vi "rsscope_core_global.vi"() -> ()   [LabVIEW 2014] (continued)
\n\nAvailable Repeated Capabilities:\nEyeDiagram: ED1, ED2, ED3, ED4\r\n\nRemote-control command(s):\nEYE<m>:HORizontal:ABSolute:POSition"}, {"Level"=5, "Class Only"=FALSE, "Identifier"="RSSCOPE_ATTR_EYE_DIAGRAM_HORIZONTAL_SETTINGS_BIT_RATE", "Descriptive Name"="Eye Diagram Horizontal Settings Bit Rate", "Data Type"=1, "Command"="EYE{EyeDiagram}:HOR:UINT:BITR", "Access"=2, "Range Table"="RsScope_rngEyeDiagramHorizontalSettingsBitRate", "Read Callback"="", "Write Callback"="", "Supported Models"="", "Instrument Options"="K91|K93", "Flags"=0, "Help"="Sets the nominal frequency or bit rate of the data signal.\n\nAvailable Repeated Capabilities:\nEyeDiagram: ED1, ED2, ED3, ED4\r\n\nRemote-control command(s):\nEYE<m>:HORizontal:UINTerval:BITRate"}, {"Level"=5, "Class Only"=FALSE, "Identifier"="RSSCOPE_ATTR_EYE_DIAGRAM_HORIZONTAL_SETTINGS_RANGE_UI", "Descriptive Name"="Eye Diagram Horizontal Settings Range UI", "Data Type"=1, "Command"="EYE{EyeDiagram}:HOR:UINT:RANG", "Access"=2, "Range Table"="RsScope_rngEyeDiagramHorizontalSettingsRangeUI", "Read Callback"="", "Write Callback"="", "Supported Models"="", "Instrument Options"="K91|K93", "Flags"=0, "Help"="Sets the number of unit intervals that are visible in the eye diagram.\n\nAvailable Repeated Capabilities:\nEyeDiagram: ED1, ED2, ED3, ED4\r\n\nRemote-control command(s):\nEYE<m>:HORizontal:UINTerval:RANGe"}, {"Level"=5, "Class Only"=FALSE, "Identifier"="RSSCOPE_ATTR_EYE_DIAGRAM_HORIZONTAL_SETTINGS_POSITION_UI", "Descriptive Name"="Eye Diagram Horizontal Settings Position UI", "Data Type"=1, "Command"="EYE{EyeDiagram}:HOR:UINT:POS", "Access"=2, "Range Table"="RsScope_rngEyeDiagramHorizontalSettingsPositionUI", "Read Callback"="", "Write Callback"="", "Supported Models"="", "Instrument Options"="K91|K93", "Flags"=0, "Help"="Sets the zero point in the diagram, in unit intervals. The zero point is the alignment point on which the segment timestamps are superimposed.\n\nAvailable Repeated Capabilities:\nEyeDiagram: ED1, ED2, ED3, ED4\r\n\nRemote-control command(s):\nEYE<m>:HORizontal:UINTerval:POSition"}, {"Level"=4, "Class Only"=TRUE, "Identifier"="", "Descriptive Name"="Display", "Data Type"=0, "Command"="", "Access"=0, "Range Table"="", "Read Callback"="", "Write Callback"="", "Supported Models"="", "Instrument Options"="", "Flags"=0, "Help"="Define the appearance of the individual eye diagram."}, {"Level"=5, "Class Only"=FALSE, "Identifier"="RSSCOPE_ATTR_EYE_DIAGRAM_MAX_SLICES_PER_ACQUISITION", "Descriptive Name"="Eye Diagram Max Slices Per Acquisition", "Data Type"=0, "Command"="EYE{EyeDiagram}:MSL", "Access"=2, "Range Table"="RsScope_rngEyeDiagramMaxSlicesPerAcquisition", "Read Callback"="", "Write Callback"="", "Supported Models"="", "Instrument Options"="K91|K93", "Flags"=0, "Help"="Sets the number of waveform slices for a single acquisition.\n\nAvailable Repeated Capabilities:\nEyeDiagram: ED1, ED2, ED3, ED4\r\n\nRemote-control command(s):\nEYE<m>:MSLices"}, {"Level"=5, "Class Only"=FALSE, "Identifier"="RSSCOPE_ATTR_EYE_DIAGRAM_EYE_STRIPE_DISPLAY_MODE", "Descriptive Name"="Eye Diagram Eye Stripe Display Mode", "Data Type"=0, "Command"="EYE{EyeDiagram}:DISP", "Access"=2, "Range Table"="RsScope_rngEyeDiagramEyeStripeDisplayMode", "Read Callback"="", "Write Callback"="", "Supported Models"="", "Instrument Options"="K91|K93", "Flags"=0, "Help"="Defines when the eye stripe is shown: always, never, or during mask tests.\n\nAvailable Repeated Capabilities:\nEyeDiagram: ED1, ED2, ED3, ED4\r\n\nRemote-control command(s):\nEYE<m>:DISPlay[:MODE]"}, {"Level"=4, "Class Only"=TRUE, "Identifier"="", "Descriptive Name"="Qualify", "Data Type"=0, "Command"="", "Access"=0, "Range Table"="", "Read Callback"="", "Write Callback"="", "Supported Models"="", "Instrument Options"="", "Flags"=0, "Help"="Restrict the slices that contribute to the eye diagram. The restriction can be in horizontal direction (gate), or in vertical direction using the reference level."}, {"Level"=5, "Class Only"=FALSE, "Identifier"="RSSCOPE_ATTR_EYE_DIAGRAM_GATE_STATE", "Descriptive Name"="Eye Diagram Gate State", "Data Type"=3, "Command"="EYE{EyeDiagram}:QUAL:GATE", "Access"=2, "Range Table"="", "Read Callback"="", "Write Callback"="", "Supported Models"="", "Instrument Options"="K91|K93", "Flags"=0, "Help"="Enables the gate.\n\nAvailable Repeated Capabilities:\nEyeDiagram: ED1, ED2, ED3, ED4\r\n\nRemote-control command(s):\nEYE<m>:QUALify:GATE[:STATe]"}, {"Level"=5, "Class Only"=FALSE, "Identifier"="RSSCOPE_ATTR_EYE_DIAGRAM_GATE_COUPLING_MODE", "Descriptive Name"="Eye Diagram Gate Coupling Mode", "Data Type"=0, "Command"="EYE{EyeDiagram}:QUAL:GATE:COUP", "Access"=2, "Range Table"="RsScope_rngEyeDiagramGateCouplingMode", "Read Callback"="", "Write Callback"="", "Supported Models"="", "Instrument Options"="K91|K93", "Flags"=0, "Help"="Sets the gate coupling. To use cursor lines or zoom areas as gate limits, the cursor or zoom must be defined before.\n\nAvailable Repeated Capabilities:\nEyeDiagram: ED1, ED2, ED3, ED4\r\n\nRemote-control command(s):\nEYE<m>:QUALify:GATE:COUPling"}, {"Level"=5, "Class Only"=FALSE, "Identifier"="RSSCOPE_ATTR_EYE_DIAGRAM_GATE_MODE", "Descriptive Name"="Eye Diagram Gate Mode", "Data Type"=0, "Command"="EYE{EyeDiagram}:QUAL:GATE:MODE", "Access"=2, "Range Table"="rsscope_rngAbsRel", "Read Callback"="", "Write Callback"="", "Supported Models"="", "Instrument Options"="K91|K93", "Flags"=0, "Help"="Defines whether the gate limit is defined in absolute or relative values when no gate coupling is set.\n\nAvailable Repeated Capabilities:\nEyeDiagram: ED1, ED2, ED3, ED4\r\n\nRemote-control command(s):\nEYE<m>:QUALify:GATE:MODE"}, {"Level"=5, "Class Only"=FALSE, "Identifier"="RSSCOPE_ATTR_EYE_DIAGRAM_GATE_ABSOLUTE_START", "Descriptive Name"="Eye Diagram Gate Absolute Start", "Data Type"=1, "Command"="EYE{EyeDiagram}:QUAL:GATE:ABS:STAR", "Access"=2, "Range Table"="", "Read Callback"="", "Write Callback"="", "Supported Models"="", "Instrument Options"="K91|K93", "Flags"=0, "Help"="Set the absolute time values for gate start.\n\nAvailable Repeated Capabilities:\nEyeDiagram: ED1, ED2, ED3, ED4\r\n\nRemote-control command(s):\nEYE<m>:QUALify:GATE:ABSolute:STARt"}, {"Level"=5, "Class Only"=FALSE, "Identifier"="RSSCOPE_ATTR_EYE_DIAGRAM_GATE_ABSOLUTE_STOP", "Descriptive Name"="Eye Diagram Gate Absolute Stop", "Data Type"=1, "Command"="EYE{EyeDiagram}:QUAL:GATE:ABS:STOP", "Access"=2, "Range Table"="", "Read Callback"="", "Write Callback"="", "Supported Models"="", "Instrument Options"="K91|K93", "Flags"=0, "Help"="Set the absolute time values for gate end.\n\nAvailable Repeated Capabilities:\nEyeDiagram: ED1, ED2, ED3, ED4\r\n\nRemote-control command(s):\nEYE<m>:QUALify:GATE:ABSolute:STOP"}, {"Level"=5, "Class Only"=FALSE, "Identifier"="RSSCOPE_ATTR_EYE_DIAGRAM_GATE_RELATIVE_START", "Descriptive Name"="Eye Diagram Gate Relative Start", "Data Type"=1, "Command"="EYE{EyeDiagram}:QUAL:GATE:REL:STAR", "Access"=2, "Range Table"="RsScope_rngPercent", "Read Callback"="", "Write Callback"="", "Supported Models"="", "Instrument Options"="K91|K93", "Flags"=0, "Help"="Set the relative values for gate start and gate end.\n\nAvailable Repeated Capabilities:\nEyeDiagram: ED1, ED2, ED3, ED4\r\n\nRemote-control command(s):\nEYE<m>:QUALify:GATE:RELative:STARt"}, {"Level"=5, "Class Only"=FALSE, "Identifier"="RSSCOPE_ATTR_EYE_DIAGRAM_GATE_RELATIVE_STOP", "Descriptive Name"="Eye Diagram Gate Relative Stop", "Data Type"=1, "Command"="EYE{EyeDiagram}:QUAL:GATE:REL:STOP", "Access"=2, "Range Table"="RsScope_rngPercent", "Read Callback"="", "Write Callback"="", "Supported Models"="", "Instrument Options"="K91|K93", "Flags"=0, "Help"="Set the relative values for gate start and gate end.\n\nAvailable Repeated Capabilities:\nEyeDiagram: ED1, ED2, ED3, ED4\r\n\nRemote-control command(s):\nEYE<m>:QUALify:GATE:RELative:STOP"}, {"Level"=5, "Class Only"=FALSE, "Identifier"="RSSCOPE_ATTR_EYE_DIAGRAM_GATE_CURSOR", "Descriptive Name"="Eye Diagram Gate Cursor", "Data Type"=0, "Command"="EYE{EyeDiagram}:QUAL:GATE:CURS", "Access"=2, "Range Table"="rsscope_rngCursor", "Read Callback"="", "Write Callback"="", "Supported Models"="", "Instrument Options"="K91|K93", "Flags"=0, "Help"="Selects the cursor set to be used for eye gating. The gate area is defined by the cursor lines.\n\nAvailable Repeated Capabilities:\nEyeDiagram: ED1, ED2, ED3, ED4\r\n\nRemote-control command(s):\nEYE<m>:QUALify:GATE:CURSor"}, {"Level"=5, "Class Only"=FALSE, "Identifier"="RSSCOPE_ATTR_EYE_DIAGRAM_SIGNAL_STATE", "Descriptive Name"="Eye Diagram Signal State", "Data Type"=3, "Command"="EYE{EyeDiagram}:QUAL:SIGN", "Access"=2, "Range Table"="", "Read Callback"="", "Write Callback"="", "Supported Models"="", "Instrument Options"="K91|K93", "Flags"=0, "Help"="Enables the waveform-based qualification for the eye generation.\n\nAvailable Repeated Capabilities:\nEyeDiagram: ED1, ED2, ED3, ED4\r\n\nRemote-control command(s):\nEYE<m>:QUALify:SIGNal[:STATe]"}, {"Level"=5, "Class Only"=FALSE, "Identifier"="RSSCOPE_ATTR_EYE_DIAGRAM_SIGNAL_SOURCE", "Descriptive Name"="Eye Diagram Signal Source", "Data Type"=0, "Command"="EYE{EyeDiagram}:QUAL:SIGN:SOUR", "Access"=2, "Range Table"="rsscope_rngEyeDiagramSource", "Read Callback"="", "Write Callback"="", "Supported Models"="", "Instrument Options"="K91|K93", "Flags"=0, "Help"="Selects the waveform to be compared.\n\nAvailable Repeated Capabilities:\nEyeDiagram: ED1, ED2, ED3, ED4\r\n\nRemote-control command(s):\nEYE<m>:QUALify:SIGNal:SOURce"}, {"Level"=5, "Class Only"=FALSE, "Identifier"="RSSCOPE_ATTR_EYE_DIAGRAM_SIGNAL_CONDITION", "Descriptive Name"="Eye Diagram Signal Condition", "Data Type"=0, "Command"="EYE{EyeDiagram}:QUAL:SIGN:COND", "Access"=2, "Range Table"="rsscope_rngEyeDiagramSignalCondition", "Read Callback"="", "Write Callback"="", "Supported Models"="", "Instrument Options"="K91|K93", "Flags"=0, "Help"="Selects the comparison condition: the waveform level must be greater or less than the threshold.\n\nAvailable Repeated Capabilities:\nEyeDiagram: ED1, ED2, ED3, ED4\r\n\nRemote-control command(s):\nEYE<m>:QUALify:SIGNal:CONDition"}, {"Level"=5, "Class Only"=FALSE, "Identifier"="RSSCOPE_ATTR_EYE_DIAGRAM_SIGNAL_VERTICAL_REFERENCE_LEVEL", "Descriptive Name"="Eye Diagram Signal Vertical Reference Level", "Data Type"=0, "Command"="EYE{EyeDiagram}:QUAL:SIGN:LSEL", "Access"=2, "Range Table"="RsScope_rngEyeDiagramVerticalReferenceLevel", "Read Callback"="", "Write Callback"="", "Supported Models"="", "Instrument Options"="K91|K93", "Flags"=0, "Help"="Selects the threshold. You can use the lower, middle, or upper reference level. These levels are the reference levels that are defined for measurements.\n\nAvailable Repeated Capabilities:\nEyeDiagram: ED1, ED2, ED3, ED4\r\n\nRemote-control command(s):\nEYE<m>:QUALify:SIGNal:LSELect"}, {"Level"=4, "Class Only"=TRUE, "Identifier"="", "Descriptive Name"="Filter", "Data Type"=0, "Command"="", "Access"=0, "Range Table"="", "Read Callback"="", "Write Callback"="", "Supported Models"="", "Instrument Options"="", "Flags"=0, "Help"="Select waveform slices for eye generation dependent on the bit status."}, {"Level"=5, "Class Only"=FALSE, "Identifier"="RSSCOPE_ATTR_EYE_DIAGRAM_FILTER_STATE", "Descriptive Name"="Eye Diagram Filter State", "Data Type"=3, "Command"="EYE{EyeDiagram}:FILT:STAT", "Access"=2, "Range Table"="", "Read Callback"="", "Write Callback"="", "Supported Models"="", "Instrument Options"="K91|K93", "Flags"=0, "Help"="Applies the filter settings to the data signal.\n\nAvailable Repeated Capabilities:\nEyeDiagram: ED1, ED2, ED3, ED4\r\n\nRemote-control command(s):\nEYE<m>:FILTer:STATe"}, {"Level"=5, "Class Only"=FALSE, "Identifier"="RSSCOPE_ATTR_EYE_DIAGRAM_FILTER_BIT_SEQUENCE_MODE", "Descriptive Name"="Eye Diagram Filter Bit Sequence Mode", "Data Type"=0, "Command"="EYE{EyeDiagram}:FILT:BPAT:MODE", "Access"=2, "Range Table"="RsScope_rngEyeDiagramFilterBitSequenceMode", "Read Callback"="", "Write Callback"="", "Supported Models"="", "Instrument Options"="K91|K93", "Flags"=0, "Help"="Selects which bits contribute to the eye generation.\n\nAvailable Repeated Capabilities:\nEyeDiagram: ED1, ED2, ED3, ED4\r\n\nRemote-control command(s):\nEYE<m>:FILTer:BPATtern:MODE"}, {"Level"=5, "Class Only"=FALSE, "Identifier"="RSSCOPE_ATTR_EYE_DIAGRAM_FILTER_PATTERN_CENTER_BIT", "Descriptive Name"="Eye Diagram Filter Pattern Center Bit", "Data Type"=0, "Command"="EYE{EyeDiagram}:FILT:BPAT:CENT", "Access"=2, "Range Table"="RsScope_rngBitState", "Read Callback"="", "Write Callback"="", "Supported Models"="", "Instrument Options"="K91|K93", "Flags"=0, "Help"="Set the values of the indicated center bits.\n\nAvailable Repeated Capabilities:\nEyeDiagram: ED1, ED2, ED3, ED4\r\n\nRemote-control command(s):\nEYE<m>:FILTer:BPATtern:CENTer"}, {"Level"=5, "Class Only"=FALSE, "Identifier"="RSSCOPE_ATTR_EYE_DIAGRAM_FILTER_PATTERN_SHIFT_BIT_LEFT", "Descriptive Name"="Eye Diagram Filter Pattern Shift Bit Left", "Data Type"=4, "Command"="EYE{EyeDiagram}:FILT:BPAT:SLEF", "Access"=1, "Range Table"="", "Read Callback"="", "Write Callback"="", "Supported Models"="", "Instrument Options"="K91|K93", "Flags"=0, "Help"="Shifts the pattern one bit to the left.\n\nAvailable Repeated Capabilities:\nEyeDiagram: ED1, ED2, ED3, ED4\r\n\nRemote-control command(s):\nEYE<m>:FILTer:BPATtern:SLEFt"}, {"Level"=5, "Class Only"=FALSE, "Identifier"="RSSCOPE_ATTR_EYE_DIAGRAM_FILTER_PATTERN_SHIFT_BIT_RIGHT", "Descriptive Name"="Eye Diagram Filter Pattern Shift Bit Right", "Data Type"=4, "Command"="EYE{EyeDiagram}:FILT:BPAT:SRIG", "Access"=1, "Range Table"="", "Read Callback"="", "Write Callback"="", "Supported Models"="", "Instrument Options"="K91|K93", "Flags"=0, "Help"="Shifts the pattern one bit to the right.\n\nAvailable Repeated Capabilities:\nEyeDiagram: ED1, ED2, ED3, ED4\r\n\nRemote-control command(s):\nEYE<m>:FILTer:BPATtern:SRIGht"}, {"Level"=5, "Class Only"=FALSE, "Identifier"="RSSCOPE_ATTR_EYE_DIAGRAM_FILTER_FRAME_TYPE", "Descriptive Name"="Eye Diagram Filter Frame Type", "Data Type"=0, "Command"="EYE{EyeDiagram}:FILT:DDR:FTYP", "Access"=2, "Range Table"="RsScope_rngEyeDiagramDDRFrameFilter", "Read Callback"="", "Write Callback"="", "Supported Models"="", "Instrument Options"="K91|K93", "Flags"=0, "Help"="Sets which frame types contribute to the eye diagram.\n\nAvailable Repeated Capabilities:\nEyeDiagram: ED1, ED2, ED3, ED4\r\n\nRemote-control command(s):\nEYE<m>:FILTer:DDR:FTYPe"}, {"Level"=5, "Class Only"=FALSE, "Identifier"="RSSCOPE_ATTR_EYE_DIAGRAM_FILTER_LENGTH_ERRORS", "Descriptive Name"="Eye Diagram Filter Length Errors", "Data Type"=3, "Command"="EYE{EyeDiagram}:FILT:DDR:LEN", "Access"=2, "Range Table"="", "Read Callback"="", "Write Callback"="", "Supported Models"="", "Instrument Options"="K91|K93", "Flags"=0, "Help"="If enabled, the length errors contribute to the eye diagram.\n\nAvailable Repeated Capabilities:\nEyeDiagram: ED1, ED2, ED3, ED4\r\n\nRemote-control command(s):\nEYE<m>:FILTer:DDR:LENerror"}, {"Level"=5, "Class Only"=FALSE, "Identifier"="RSSCOPE_ATTR_EYE_DIAGRAM_FILTER_RESET", "Descriptive Name"="Eye Diagram Filter Reset", "Data Type"=4, "Command"="EYE{EyeDiagram}:FILT:BPAT:RES", "Access"=1, "Range Table"="", "Read Callback"="", "Write Callback"="", "Supported Models"="", "Instrument Options"="K91|K93", "Flags"=0, "Help"="Resets the bit sequence filter to the default (DC for all bits).\n\nAvailable Repeated Capabilities:\nEyeDiagram: ED1, ED2, ED3, ED4\r\n\nRemote-control command(s):\nEYE<m>:FILTer:BPATtern:RESet"}, {"Level"=4, "Class Only"=TRUE, "Identifier"="", "Descriptive Name"="Results of Mask Tests", "Data Type"=0, "Command"="", "Access"=0, "Range Table"="", "Read Callback"="", "Write Callback"="", "Supported Models"="", "Instrument Options"="", "Flags"=0, "Help"="Mask tests on eye diagrams"}, {"Level"=5, "Class Only"=FALSE, "Identifier"="RSSCOPE_ATTR_EYE_DIAGRAM_MASK_TESTS_SLICES_COMPLETED", "Descriptive Name"="Eye Diagram Mask Tests Slices Completed", "Data Type"=0, "Command"="MTES:RES:COUN:SLIC?", "Access"=0, "Range Table"="", "Read Callback"="rsscope_formatMaskNameInt32_ReadCallback.vi", "Write Callback"="", "Supported Models"="", "Instrument Options"="K91|K93", "Flags"=0, "Help"="Returns the number of slices that contributed to the eye diagram.\n\nAvailable Repeated Capabilities:\nNone\n\nRemote-control command(s):\nMTESt:RESult:COUNt:SLICes?"}, {"Level"=5, "Class Only"=FALSE, "Identifier"="RSSCOPE_ATTR_EYE_DIAGRAM_MASK_TESTS_SLICE_HITS", "Descriptive Name"="Eye Diagram Mask Tests Slice Hits", "Data Type"=0, "Command"="MTES:RES:COUN:FSL?", "Access"=0, "Range Table"="", "Read Callback"="rsscope_formatMaskNameInt32_ReadCallback.vi", "Write Callback"="", "Supported Models"="", "Instrument Options"="K91|K93", "Flags"=0, "Help"="Returns the number of slices that violated the mask.\n\nAvailable Repeated Capabilities:\nNone\n\nRemote-control command(s):\nMTESt:RESult:COUNt:FSLices?"}, {"Level"=5, "Class Only"=FALSE, "Identifier"="RSSCOPE_ATTR_EYE_DIAGRAM_MASK_TESTS_VIOLATION_INDEX", "Descriptive Name"="Eye Diagram Mask Tests Violation Index", "Data Type"=0, "Command"="", "Access"=2, "Range Table"="", "Read Callback"="", "Write Callback"="", "Supported Models"="", "Instrument Options"="K91|K93", "Flags"=0, "Help"="Sets selector repeated capability Violation. Corresponds to the number in the &apos;Violation&apos; column of mask test result.\n\nAvailable Repeated Capabilities:\nNone\n\nRemote-control command(s):\n"}, {"Level"=5, "Class Only"=FALSE, "Identifier"="RSSCOPE_ATTR_EYE_DIAGRAM_MASK_TESTS_VIOLATION_COUNT", "Descriptive Name"="Eye Diagram Mask Tests Violation Count", "Data Type"=0, "Command"="MTES:RES:VIOL<Violation>:COUN?", "Access"=0, "Range Table"="", "Read Callback"="rsscope_formatMaskNameViolationInt32_ReadCallback.vi", "Write Callback"="", "Supported Models"="", "Instrument Options"="K91|K93", "Flags"=0, "Help"="Returns the count of violations of mask test result.\n\nAvailable Repeated Capabilities:\nNone\n\nRemote-control command(s):\nMTESt:RESult:VIOLation<m>:COUNt?"}, {"Level"=5, "Class Only"=FALSE, "Identifier"="RSSCOPE_ATTR_EYE_DIAGRAM_MASK_TESTS_VIOLATION_START_TIME", "Descriptive Name"="Eye Diagram Mask Tests Violation Start Time", "Data Type"=1, "Command"="MTES:RES:VIOL<Violation>:STAR?", "Access"=0, "Range Table"="", "Read Callback"="rsscope_formatMaskNameViolationReal64_ReadCallback.vi", "Write Callback"="", "Supported Models"="", "Instrument Options"="K91|K93", "Flags"=0, "Help"="Return the start time of the slice with the indicated violation.\n\nAvailable Repeated Capabilities:\nNone\n\nRemote-control command(s):\nMTESt:RESult:VIOLation<m>:STARt?"}, {"Level"=5, "Class Only"=FALSE, "Identifier"="RSSCOPE_ATTR_EYE_DIAGRAM_MASK_TESTS_VIOLATION_STOP_TIME", "Descriptive Name"="Eye Diagram Mask Tests Violation Stop Time", "Data Type"=1, "Command"="MTES:RES:VIOL<Violation>:STOP?", "Access"=0, "Range Table"="", "Read Callback"="rsscope_formatMaskNameViolationReal64_ReadCallback.vi", "Write Callback"="", "Supported Models"="", "Instrument Options"="K91|K93", "Flags"=0, "Help"="Return the stop time of the slice with the indicated violation.\n\nAvailable Repeated Capabilities:\nNone\n\nRemote-control command(s):\nMTESt:RESult:VIOLation<m>:STOP?"}, {"Level"=5, "Class Only"=FALSE, "Identifier"="RSSCOPE_ATTR_EYE_DIAGRAM_MASK_TESTS_VIOLATION_SLICE", "Descriptive Name"="Eye Diagram Mask Tests Violation Slice", "Data Type"=0, "Command"="MTES:RES:VIOL<Violation>?", "Access"=0, "Range Table"="", "Read Callback"="rsscope_formatMaskNameViolationInt32_ReadCallback.vi", "Write Callback"="", "Supported Models"="", "Instrument Options"="K91|K93", "Flags"=0, "Help"="Returns the slice at the violation of mask test result.\n\nAvailable Repeated Capabilities:\nNone\n\nRemote-control command(s):\nMTESt:RESult:VIOLation<m>[:SLICe]?"}, {"Level"=2, "Class Only"=TRUE, "Identifier"="", "Descriptive Name"="100BASE-T1", "Data Type"=0, "Command"="", "Access"=0, "Range Table"="", "Read Callback"="", "Write Callback"="", "Supported Models"="", "Instrument Options"="", "Flags"=0, "Help"="This class contains attributes that configure the Ethernet protocol 100BASE-T1.\n\nAttributes in this class require option R&S RTO-K57."}, {"Level"=3, "Class Only"=FALSE, "Identifier"="RSSCOPE_ATTR_PROTOCOL_100BASE_T1_ATTENUATION", "Descriptive Name"="Protocol 100BASE-T1 Attenuation", "Data Type"=1, "Command"="BUS{SerialBus}:HBTO:ATTN", "Access"=2, "Range Table"="RsScope_rngProtocol100BASE_T1Attenuation", "Read Callback"="", "Write Callback"="", "Supported Models"="", "Instrument Options"="K57", "Flags"=0, "Help"="Sets the attenuation factor. It is used to de-amplify the reverse signal before subtracting it from the forward signal.\n\nAvailable Repeated Capabilities:\nSerialBus: SB1, SB2, SB3, SB4\r\n\nRemote-control command(s):\nBUS<m>:HBTO:ATTN"}, {"Level"=3, "Class Only"=FALSE, "Identifier"="RSSCOPE_ATTR_PROTOCOL_100BASE_T1_FORWARD_POSITIVE_SOURCE", "Descriptive Name"="Protocol 100BASE-T1 Forward Positive Source", "Data Type"=0, "Command"="BUS{SerialBus}:HBTO:FDAP", "Access"=2, "Range Table"="rsscope_rngProtocolDataSource", "Read Callback"="", "Write Callback"="", "Supported Models"="", "Instrument Options"="K57", "Flags"=0, "Help"="Selects the DA+ source of the provided forward single ended signal, if RSSCOPE_ATTR_PROTOCOL_100BASE_T1_FORWARD_SIGNAL_TYPE is set to Single.\n\nAvailable Repeated Capabilities:\nSerialBus: SB1, SB2, SB3, SB4\r\n\nRemote-control command(s):\nBUS<m>:HBTO:FDAP"}, {"Level"=3, "Class Only"=FALSE, "Identifier"="RSSCOPE_ATTR_PROTOCOL_100BASE_T1_FORWARD_NEGATIVE_SOURCE", "Descriptive Name"="Protocol 100BASE-T1 Forward Negative Source", "Data Type"=0, "Command"="BUS{SerialBus}:HBTO:FDAM", "Access"=2, "Range Table"="rsscope_rngProtocolDataSource", "Read Callback"="", "Write Callback"="", "Supported Models"="", "Instrument Options"="K57", "Flags"=0, "Help"="Selects the DA- source of the provided forward single ended signal, if RSSCOPE_ATTR_PROTOCOL_100BASE_T1_FORWARD_SIGNAL_TYPE is set to Single.\n\nAvailable Repeated Capabilities:\nSerialBus: SB1, SB2, SB3, SB4\r\n\nRemote-control command(s):\nBUS<m>:HBTO:FDAM"}, {"Level"=3, "Class Only"=FALSE, "Identifier"="RSSCOPE_ATTR_PROTOCOL_100BASE_T1_FORWARD_DIFFERENTIAL_SOURCE", "Descriptive Name"="Protocol 100BASE-T1 Forward Differential Source", "Data Type"=0, "Command"="BUS{SerialBus}:HBTO:FDIF", "Access"=2, "Range Table"="rsscope_rngProtocolDataSource", "Read Callback"="", "Write Callback"="", "Supported Models"="", "Instrument Options"="K57", "Flags"=0, "Help"="Sets the source of the provided forward differential signal, if RSSCOPE_ATTR_PROTOCOL_100BASE_T1_FORWARD_SIGNAL_TYPE is set to Differential.\n\nAvailable Repeated Capabilities:\nSerialBus: SB1, SB2, SB3, SB4\r\n\nRemote-control command(s):\nBUS<m>:HBTO:FDIF"}, {"Level"=3, "Class Only"=FALSE, "Identifier"="RSSCOPE_ATTR_PROTOCOL_100BASE_T1_FORWARD_SIGNAL_TYPE", "Descriptive Name"="Protocol 100BASE-T1 Forward Signal Type", "Data Type"=0, "Command"="BUS{SerialBus}:HBTO:FTYP", "Access"=2, "Range Table"="RsScope_rngSignalType", "Read Callback"="", "Write Callback"="", "Supported Models"="", "Instrument Options"="K57", "Flags"=0, "Help"="Sets the type of forward signal measurement.\n\nAvailable Repeated Capabilities:\nSerialBus: SB1, SB2, SB3, SB4\r\n\nRemote-control command(s):\nBUS<m>:HBTO:FTYP"}, {"Level"=3, "Class Only"=FALSE, "Identifier"="RSSCOPE_ATTR_PROTOCOL_100BASE_T1_REVERSE_POSITIVE_SOURCE", "Descriptive Name"="Protocol 100BASE-T1 Reverse Positive Source", "Data Type"=0, "Command"="BUS{SerialBus}:HBTO:RDAP", "Access"=2, "Range Table"="rsscope_rngProtocolDataSource", "Read Callback"="", "Write Callback"="", "Supported Models"="", "Instrument Options"="K57", "Flags"=0, "Help"="Selects the DA+ source of the provided reversed single ended signal, if RSSCOPE_ATTR_PROTOCOL_100BASE_T1_REVERSE_SIGNAL_TYPE is set to Single.\n\nAvailable Repeated Capabilities:\nSerialBus: SB1, SB2, SB3, SB4\r\n\nRemote-control command(s):\nBUS<m>:HBTO:RDAP"}, {"Level"=3, "Class Only"=FALSE, "Identifier"="RSSCOPE_ATTR_PROTOCOL_100BASE_T1_REVERSE_NEGATIVE_SOURCE", "Descriptive Name"="Protocol 100BASE-T1 Reverse Negative Source", "Data Type"=0, "Command"="BUS{SerialBus}:HBTO:RDAM", "Access"=2, "Range Table"="rsscope_rngProtocolDataSource", "Read Callback"="", "Write Callback"="", "Supported Models"="", "Instrument Options"="K57", "Flags"=0, "Help"="Selects the DA- source of the provided reversed single ended signal, if RSSCOPE_ATTR_PROTOCOL_100BASE_T1_REVERSE_SIGNAL_TYPE is set to Single.\n\nAvailable Repeated Capabilities:\nSerialBus: SB1, SB2, SB3, SB4\r\n\nRemote-control command(s):\nBUS<m>:HBTO:RDAM"}, {"Level"=3, "Class Only"=FALSE, "Identifier"="RSSCOPE_ATTR_PROTOCOL_100BASE_T1_REVERSE_DIFFERENTIAL_SOURCE", "Descriptive Name"="Protocol 100BASE-T1 Reverse Differential Source", "Data Type"=0, "Command"="BUS{SerialBus}:HBTO:RDIF", "Access"=2, "Range Table"="rsscope_rngProtocolDataSource", "Read Callback"="", "Write Callback"="", "Supported Models"="", "Instrument Options"="K57", "Flags"=0, "Help"="Sets the source of the provided reversed differential signal, if RSSCOPE_ATTR_PROTOCOL_100BASE_T1_REVERSE_SIGNAL_TYPE is set to Differential.\n\nAvailable Repeated Capabilities:\nSerialBus: SB1, SB2, SB3, SB4\r\n\nRemote-control command(s):\nBUS<m>:HBTO:RDIF"}, {"Level"=3, "Class Only"=FALSE, "Identifier"="RSSCOPE_ATTR_PROTOCOL_100BASE_T1_REVERSE_SIGNAL_TYPE", "Descriptive Name"="Protocol 100BASE-T1 Reverse Signal Type", "Data Type"=0, "Command"="BUS{SerialBus}:HBTO:RTYP", "Access"=2, "Range Table"="RsScope_rngSignalReverseType", "Read Callback"="", "Write Callback"="", "Supported Models"="", "Instrument Options"="K57", "Flags"=0, "Help"="Sets the type of reverse signal measurement.\n\nAvailable Repeated Capabilities:\nSerialBus: SB1, SB2, SB3, SB4\r\n\nRemote-control command(s):\nBUS<m>:HBTO:RTYP"}, {"Level"=3, "Class Only"=FALSE, "Identifier"="RSSCOPE_ATTR_PROTOCOL_100BASE_T1_POLARITY", "Descriptive Name"="Protocol 100BASE-T1 Polarity", "Data Type"=0, "Command"="BUS{SerialBus}:HBTO:POL", "Access"=2, "Range Table"="rsscope_rngEthernetPolarity", "Read Callback"="", "Write Callback"="", "Supported Models"="", "Instrument Options"="K57", "Flags"=0, "Help"="Selects the polarity of the data signal.\n\nAvailable Repeated Capabilities:\nSerialBus: SB1, SB2, SB3, SB4\r\n\nRemote-control command(s):\nBUS<m>:HBTO:POLarity"}, {"Level"=3, "Class Only"=FALSE, "Identifier"="RSSCOPE_ATTR_PROTOCOL_100BASE_T1_THRESHOLD", "Descriptive Name"="Protocol 100BASE-T1 Threshold", "Data Type"=1, "Command"="BUS{SerialBus}:HBTO:THR", "Access"=2, "Range Table"="RsScope_rngProtocol100BASE_T1Threshold", "Read Callback"="", "Write Callback"="", "Supported Models"="", "Instrument Options"="K57", "Flags"=0, "Help"="Sets an user-defined threshold value.\n\nAvailable Repeated Capabilities:\nSerialBus: SB1, SB2, SB3, SB4\r\n\nRemote-control command(s):\nBUS<m>:HBTO:THReshold"}, {"Level"=3, "Class Only"=FALSE, "Identifier"="RSSCOPE_ATTR_PROTOCOL_100BASE_T1_MODE", "Descriptive Name"="Protocol 100BASE-T1 Mode", "Data Type"=0, "Command"="BUS{SerialBus}:HBTO:MODE", "Access"=2, "Range Table"="RsScope_rngSignalDirection", "Read Callback"="", "Write Callback"="", "Supported Models"="", "Instrument Options"="K57", "Flags"=0, "Help"="Selects the direction of the full-duplex signal you want to look at.\n\nAvailable Repeated Capabilities:\nSerialBus: SB1, SB2, SB3, SB4\r\n\nRemote-control command(s):\nBUS<m>:HBTO:MODE"}, {"Level"=3, "Class Only"=FALSE, "Identifier"="RSSCOPE_ATTR_PROTOCOL_100BASE_T1_SYMBOL_RATE", "Descriptive Name"="Protocol 100BASE-T1 Symbol Rate", "Data Type"=1, "Command"="BUS{SerialBus}:HBTO:SYMR", "Access"=2, "Range Table"="RsScope_rngProtocol100BASE_T1SymbolRate", "Read Callback"="", "Write Callback"="", "Supported Models"="", "Instrument Options"="K57", "Flags"=0, "Help"="Defines the rate of ternary symbols.\n\nAvailable Repeated Capabilities:\nSerialBus: SB1, SB2, SB3, SB4\r\n\nRemote-control command(s):\nBUS<m>:HBTO:SYMRate"}, {"Level"=3, "Class Only"=TRUE, "Identifier"="", "Descriptive Name"="Decoding Results", "Data Type"=0, "Command"="", "Access"=0, "Range Table"="", "Read Callback"="", "Write Callback"="", "Supported Models"="", "Instrument Options"="", "Flags"=0, "Help"="Returns the 100BASE-T1 decoding results."}, {"Level"=4, "Class Only"=FALSE, "Identifier"="RSSCOPE_ATTR_PROTOCOL_100BASE_T1_FRAME_COUNT", "Descriptive Name"="Protocol 100BASE-T1 Frame Count", "Data Type"=0, "Command"="BUS{SerialBus}:HBTO:RES:FCO?", "Access"=0, "Range Table"="", "Read Callback"="", "Write Callback"="", "Supported Models"="", "Instrument Options"="K57", "Flags"=0, "Help"="Returns the number of decoded frames.\n\nAvailable Repeated Capabilities:\nSerialBus: SB1, SB2, SB3, SB4\r\n\nRemote-control command(s):\nBUS<m>:HBTO:RESult:FCOunt?"}, {"Level"=4, "Class Only"=FALSE, "Identifier"="RSSCOPE_ATTR_PROTOCOL_100BASE_T1_SELECTED_FRAME", "Descriptive Name"="Protocol 100BASE-T1 Selected Frame", "Data Type"=0, "Command"="", "Access"=2, "Range Table"="", "Read Callback"="", "Write Callback"="", "Supported Models"="", "Instrument Options"="", "Flags"=0, "Help"="Sets selector repeated capability Frame.\n\nAvailable Repeated Capabilities:\nNone\n\nRemote-control command(s):\n"}, {"Level"=4, "Class Only"=FALSE, "Identifier"="RSSCOPE_ATTR_PROTOCOL_100BASE_T1_FRAME_STATUS", "Descriptive Name"="Protocol 100BASE-T1 Frame Status", "Data Type"=0, "Command"="BUS{SerialBus}:HBTO:RES:FRAM<Frame>:STAT?", "Access"=0, "Range Table"="rsscope_rngProtocol100BASE_T1FrameStatus", "Read Callback"="rsscope_Format100BASE_T1FrameRepCapInt32_ReadCallback.vi", "Write Callback"="", "Supported Models"="", "Instrument Options"="K57", "Flags"=0, "Help"="Returns the state of the frame.\n\nAvailable Repeated Capabilities:\nSerialBus: SB1, SB2, SB3, SB4\r\n\nRemote-control command(s):\nBUS<m>:HBTO:RESult:FRAMe<n>:STATe?"}, {"Level"=4, "Class Only"=FALSE, "Identifier"="RSSCOPE_ATTR_PROTOCOL_100BASE_T1_FRAME_START_TIME", "Descriptive Name"="Protocol 100BASE-T1 Frame Start Time", "Data Type"=1, "Command"="BUS{SerialBus}:HBTO:RES:FRAM<Frame>:STAR?", "Access"=0, "Range Table"="", "Read Callback"="rsscope_Format100BASE_T1FrameRepCapReal64_ReadCallback.vi", "Write Callback"="", "Supported Models"="", "Instrument Options"="K57", "Flags"=0, "Help"="Returns the start time of the selected frame.\n\nAvailable Repeated Capabilities:\nSerialBus: SB1, SB2, SB3, SB4\r\n\nRemote-control command(s):\nBUS<m>:HBTO:RESult:FRAMe<n>:STARt?"}, {"Level"=4, "Class Only"=FALSE, "Identifier"="RSSCOPE_ATTR_PROTOCOL_100BASE_T1_FRAME_STOP_TIME", "Descriptive Name"="Protocol 100BASE-T1 Frame Stop Time", "Data Type"=1, "Command"="BUS{SerialBus}:HBTO:RES:FRAM<Frame>:STOP?", "Access"=0, "Range Table"="", "Read Callback"="rsscope_Format100BASE_T1FrameRepCapReal64_ReadCallback.vi", "Write Callback"="", "Supported Models"="", "Instrument Options"="K57", "Flags"=0, "Help"="Returns the end time of the selected frame.\n\nAvailable Repeated Capabilities:\nSerialBus: SB1, SB2, SB3, SB4\r\n\nRemote-control command(s):\nBUS<m>:HBTO:RESult:FRAMe<n>:STOP?"}, {"Level"=4, "Class Only"=FALSE, "Identifier"="RSSCOPE_ATTR_PROTOCOL_100BASE_T1_FRAME_LENGTH", "Descriptive Name"="Protocol 100BASE-T1 Frame Length", "Data Type"=0, "Command"="BUS{SerialBus}:HBTO:RES:FRAM<Frame>:TYPE?", "Access"=0, "Range Table"="", "Read Callback"="rsscope_Format100BASE_T1FrameRepCapInt32_ReadCallback.vi", "Write Callback"="", "Supported Models"="", "Instrument Options"="K57", "Flags"=0, "Help"="Returns the value of length / type field of the selected frame.\n\nAvailable Repeated Capabilities:\nSerialBus: SB1, SB2, SB3, SB4\r\n\nRemote-control command(s):\nBUS<m>:HBTO:RESult:FRAMe<n>:TYPE?"}, {"Level"=4, "Class Only"=FALSE, "Identifier"="RSSCOPE_ATTR_PROTOCOL_100BASE_T1_FRAME_CRC", "Descriptive Name"="Protocol 100BASE-T1 Frame CRC", "Data Type"=5, "Command"="BUS{SerialBus}:HBTO:RES:FRAM<Frame>:CRC?", "Access"=0, "Range Table"="", "Read Callback"="rsscope_Format100BASE_T1FrameRepCapInt64_ReadCallback.vi", "Write Callback"="", "Supported Models"="", "Instrument Options"="K57", "Flags"=0, "Help"="Returns the CRC (frame check) checksum of the selected frame.\n\nAvailable Repeated Capabilities:\nSerialBus: SB1, SB2, SB3, SB4\r\n\nRemote-control command(s):\nBUS<m>:HBTO:RESult:FRAMe<n>:CRC?"}, {"Level"=4, "Class Only"=FALSE, "Identifier"="RSSCOPE_ATTR_PROTOCOL_100BASE_T1_FRAME_DESTINATION", "Descriptive Name"="Protocol 100BASE-T1 Frame Destination", "Data Type"=2, "Command"="BUS{SerialBus}:HBTO:RES:FRAM<Frame>:DEST?", "Access"=0, "Range Table"="", "Read Callback"="rsscope_Format100BASE_T1FrameRepCapString_ReadCallback.vi", "Write Callback"="", "Supported Models"="", "Instrument Options"="K57", "Flags"=0, "Help"="Returns the destination address of the selected frame.\n\nAvailable Repeated Capabilities:\nSerialBus: SB1, SB2, SB3, SB4\r\n\nRemote-control command(s):\nBUS<m>:HBTO:RESult:FRAMe<n>:DESTaddress?"}, {"Level"=4, "Class Only"=FALSE, "Identifier"="RSSCOPE_ATTR_PROTOCOL_100BASE_T1_FRAME_SOURCE", "Descriptive Name"="Protocol 100BASE-T1 Frame Source", "Data Type"=2, "Command"="BUS{SerialBus}:HBTO:RES:FRAM<Frame>:SRC?", "Access"=0, "Range Table"="", "Read Callback"="rsscope_Format100BASE_T1FrameRepCapString_ReadCallback.vi", "Write Callback"="", "Supported Models"="", "Instrument Options"="K57", "Flags"=0, "Help"="Returns the source address of the selected frame.\n\nAvailable Repeated Capabilities:\nSerialBus: SB1, SB2, SB3, SB4\r\n\nRemote-control command(s):\nBUS<m>:HBTO:RESult:FRAMe<n>:SRCaddress?"}, {"Level"=4, "Class Only"=FALSE, "Identifier"="RSSCOPE_ATTR_PROTOCOL_100BASE_T1_FRAME_DESTINATION_LABEL", "Descriptive Name"="Protocol 100BASE-T1 Frame Destination Label", "Data Type"=2, "Command"="BUS{SerialBus}:HBTO:RES:FRAM<Frame>:DSYM?", "Access"=0, "Range Table"="", "Read Callback"="rsscope_Format100BASE_T1FrameRepCapString_ReadCallback.vi", "Write Callback"="", "Supported Models"="", "Instrument Options"="K57", "Flags"=0, "Help"="Returns the destination symbols of the selected frame.\n\nAvailable Repeated Capabilities:\nSerialBus: SB1, SB2, SB3, SB4\r\n\nRemote-control command(s):\nBUS<m>:HBTO:RESult:FRAMe<n>:DSYMbol?"}, {"Level"=4, "Class Only"=FALSE, "Identifier"="RSSCOPE_ATTR_PROTOCOL_100BASE_T1_FRAME_SOURCE_LABEL", "Descriptive Name"="Protocol 100BASE-T1 Frame Source Label", "Data Type"=2, "Command"="BUS{SerialBus}:HBTO:RES:FRAM<Frame>:SSYM?", "Access"=0, "Range Table"="", "Read Callback"="rsscope_Format100BASE_T1FrameRepCapString_ReadCallback.vi", "Write Callback"="", "Supported Models"="", "Instrument Options"="K57", "Flags"=0, "Help"="Returns the source symbols of the selected frame.\n\nAvailable Repeated Capabilities:\nSerialBus: SB1, SB2, SB3, SB4\r\n\nRemote-control command(s):\nBUS<m>:HBTO:RESult:FRAMe<n>:SSYMbol?"}, {"Level"=4, "Class Only"=FALSE, "Identifier"="RSSCOPE_ATTR_PROTOCOL_100BASE_T1_FRAME_BIT_RATE", "Descriptive Name"="Protocol 100BASE-T1 Frame Bit Rate", "Data Type"=5, "Command"="BUS{SerialBus}:HBTO:RES:FRAM<Frame>:BITR?", "Access"=0, "Range Table"="", "Read Callback"="rsscope_Format100BASE_T1FrameRepCapInt64_ReadCallback.vi", "Write Callback"="", "Supported Models"="", "Instrument Options"="K57", "Flags"=0, "Help"="Returns the primary bit rate.\n\nAvailable Repeated Capabilities:\nSerialBus: SB1, SB2, SB3, SB4\r\n\nRemote-control command(s):\nBUS<m>:HBTO:RESult:FRAMe<n>:BITRate?"}, {"Level"=4, "Class Only"=FALSE, "Identifier"="RSSCOPE_ATTR_PROTOCOL_100BASE_T1_FRAME_TYPE", "Descriptive Name"="Protocol 100BASE-T1 Frame Type", "Data Type"=0, "Command"="BUS{SerialBus}:HBTO:RES:FRAM<Frame>:FTYP?", "Access"=0, "Range Table"="RsScope_rngProtocol100BASE_T1FrameType", "Read Callback"="rsscope_Format100BASE_T1FrameRepCapInt32_ReadCallback.vi", "Write Callback"="", "Supported Models"="", "Instrument Options"="K57", "Flags"=0, "Help"="Returns the type of frame for the selected frame.\n\nAvailable Repeated Capabilities:\nSerialBus: SB1, SB2, SB3, SB4\r\n\nRemote-control command(s):\nBUS<m>:HBTO:RESult:FRAMe<n>:FTYPe?"}, {"Level"=4, "Class Only"=FALSE, "Identifier"="RSSCOPE_ATTR_PROTOCOL_100BASE_T1_FRAME_NUMBER_OF_WORDS", "Descriptive Name"="Protocol 100BASE-T1 Frame Number Of Words", "Data Type"=5, "Command"="BUS{SerialBus}:HBTO:RES:FRAM<Frame>:NUMW?", "Access"=0, "Range Table"="", "Read Callback"="rsscope_Format100BASE_T1FrameRepCapInt64_ReadCallback.vi", "Write Callback"="", "Supported Models"="", "Instrument Options"="K57", "Flags"=0, "Help"="Returns the number of decoded words for the selected frame.\n\nAvailable Repeated Capabilities:\nSerialBus: SB1, SB2, SB3, SB4\r\n\nRemote-control command(s):\nBUS<m>:HBTO:RESult:FRAMe<n>:NUMWords?"}, {"Level"=4, "Class Only"=FALSE, "Identifier"="RSSCOPE_ATTR_PROTOCOL_100BASE_T1_SELECTED_WORD", "Descriptive Name"="Protocol 100BASE-T1 Selected Word", "Data Type"=5, "Command"="", "Access"=2, "Range Table"="", "Read Callback"="", "Write Callback"="", "Supported Models"="", "Instrument Options"="", "Flags"=0, "Help"="Sets selector repeated capability Word.\n\nAvailable Repeated Capabilities:\nNone\n\nRemote-control command(s):\n"}, {"Level"=4, "Class Only"=FALSE, "Identifier"="RSSCOPE_ATTR_PROTOCOL_100BASE_T1_FRAME_WORD_TYPE", "Descriptive Name"="Protocol 100BASE-T1 Frame Word Type", "Data Type"=2, "Command"="BUS{SerialBus}:HBTO:RES:FRAM<Frame>:WORD<Word>:TYPE?", "Access"=0, "Range Table"="", "Read Callback"="rsscope_Format100BASE_T1WordRepCapString_ReadCallback.vi", "Write Callback"="", "Supported Models"="", "Instrument Options"="K57", "Flags"=0, "Help"="Returns the data type for the selected word.\n\nAvailable Repeated Capabilities:\nSerialBus: SB1, SB2, SB3, SB4\r\n\nRemote-control command(s):\nBUS<m>:HBTO:RESult:FRAMe<n>:WORD<o>:TYPE?"}, {"Level"=4, "Class Only"=FALSE, "Identifier"="RSSCOPE_ATTR_PROTOCOL_100BASE_T1_FRAME_WORD_VALUE", "Descriptive Name"="Protocol 100BASE-T1 Frame Word Value", "Data Type"=0, "Command"="BUS{SerialBus}:HBTO:RES:FRAM<Frame>:WORD<Word>:VAL?", "Access"=0, "Range Table"="", "Read Callback"="rsscope_Format100BASE_T1WordRepCapInt32_ReadCallback.vi", "Write Callback"="", "Supported Models"="", "Instrument Options"="K57", "Flags"=0, "Help"="Returns the data value for the selected word.\n\nAvailable Repeated Capabilities:\nSerialBus: SB1, SB2, SB3, SB4\r\n\nRemote-control command(s):\nBUS<m>:HBTO:RESult:FRAMe<n>:WORD<o>:VALue?"}, {"Level"=4, "Class Only"=FALSE, "Identifier"="RSSCOPE_ATTR_PROTOCOL_100BASE_T1_FRAME_WORD_STRING_VALUE", "Descriptive Name"="Protocol 100BASE-T1 Frame Word String Value", "Data Type"=2, "Command"="BUS{SerialBus}:HBTO:RES:FRAM<Frame>:WORD<Word>:VSTR?", "Access"=0, "Range Table"="", "Read Callback"="rsscope_Format100BASE_T1WordRepCapString_ReadCallback.vi", "Write Callback"="", "Supported Models"="", "Instrument Options"="K57", "Flags"=0, "Help"="Returns the string equivalent of data value for the selected cell.\n\nAvailable Repeated Capabilities:\nSerialBus: SB1, SB2, SB3, SB4\r\n\nRemote-control command(s):\nBUS<m>:HBTO:RESult:FRAMe<n>:WORD<o>:VSTR?"}, {"Level"=2, "Class Only"=TRUE, "Identifier"="", "Descriptive Name"="1000BASE-T1", "Data Type"=0, "Command"="", "Access"=0, "Range Table"="", "Read Callback"="", "Write Callback"="", "Supported Models"="", "Instrument Options"="", "Flags"=0, "Help"="1000BASE-T1 is a single pair Ethernet based protocol specialized for the needs of the\nautomotive industry, specified in IEEE P802.3bp.\n\nAttributes in this class require option K58."}, {"Level"=3, "Class Only"=FALSE, "Identifier"="RSSCOPE_ATTR_PROTOCOL_1000BASE_T1_REVERSE_SIGNAL_TYPE", "Descriptive Name"="Protocol 1000BASE-T1 Reverse Signal Type", "Data Type"=0, "Command"="BUS{SerialBus}:TBTO:RTYP", "Access"=2, "Range Table"="RsScope_rngSignalReverseType", "Read Callback"="", "Write Callback"="", "Supported Models"="", "Instrument Options"="K58", "Flags"=0, "Help"="Sets the type of reverse signal measurement.\n\nAvailable Repeated Capabilities:\nSerialBus: SB1, SB2, SB3, SB4\r\n\nRemote-control command(s):\nBUS<m>:TBTO:RTYP"}, 
